vi "create.vi"(6 "enqueue (back)":T1, 7 "auto-reset? (T)":bool=TRUE, 8 "error in (no error)":errorcluster, 9 "interval (1000 ms)":u32=1000, 10 "message (\"\"=Ignore)":string, 11 "destination queue":refnum<queue>) -> (0 "error out":errorcluster, 3 "timer":refnum<class "rytimer.lvclass">)   [LabVIEW 2017, in "rytimer.lvclass"]
uses:
  rytimer.lvclass
  enqueue.ctl
  rytimer.lvclass/rytimer.ctl
  daemon.vi
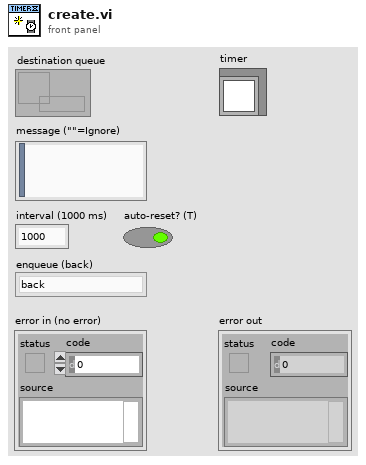
[diagram p1: front panel]
types:
  T1 = typedef "rytimer.lvclass/enqueue.ctl" = enum8{"back", "front", "back_if_absent", "front_if_absent"}
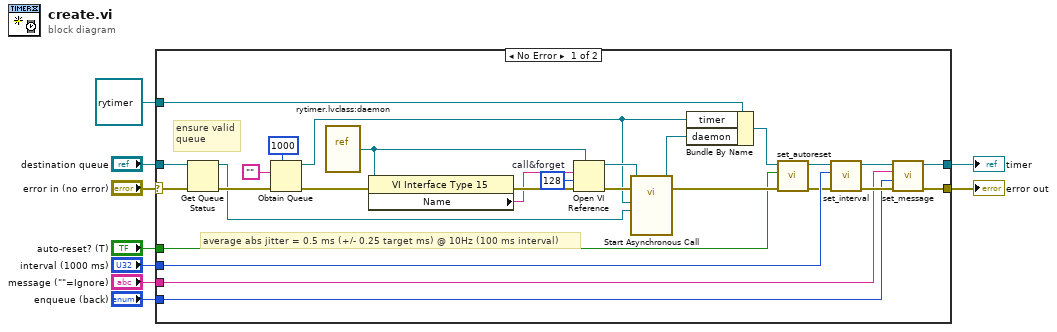
[diagram p0: block diagram]
diagram:
  n1 = case shown="No Error" "error in (no error)" {
    selector: "error in (no error)" -> [w36 w39]
    tunnel: refnum<class "rytimer.lvclass"> refnum ("timer") -> [w27 w38]
    tunnel: "interval (1000 ms)" -> [w25 _]
    tunnel: [w23 w39] -> w6
    tunnel: [w21 w38] -> w5
    tunnel: "message (\"\"=Ignore)" -> [w20 _]
    tunnel: "enqueue (back)" -> [w19 _]
    tunnel: "auto-reset? (T)" -> [w13 _]
    tunnel: "destination queue" -> [w11 _]
    frame No Error {
      w32 = 128  # call&forget
      # "average abs jitter = 0.5 ms (+/- 0.25 target ms) @ 10Hz (100 ms interval)"
      # "ensure valid\nqueue"
      n2 = Get Queue Status(queue=w11, error in (no error)=w36) -> (queue out=w10:refnum<queue>, error out=w12:errorcluster)  [unwired: 1 in, 6 out]
      n3 = Obtain Queue(max queue size (-1, unlimited)=1000, element data type="" ("Empty String Constant"), error in (no error)=w12) -> (queue out=w26:refnum<queue>, error out=w35:errorcluster)  [unwired: 2 in, 1 out]
      n4 = vi-ref "rytimer.lvclass:daemon.vi"() -> (w29:refnum<vi>)
      n5 = property class="VI Interface Type 15"(reference=w29, error in=w35) -> (error out=w34:errorcluster, "Name"=w33:string)  [unwired: 1 out]
      n6 = Open VI Reference(type specifier VI Refnum (for type only)=w29, vi path=w33, options=w32, error in (no error)=w34) -> (vi reference=w30:refnum<vi>, error out=w31:errorcluster)  [unwired: 2 in]
      n7 = call-by-ref "Start Asynchronous Call"(reference=w30, error in=w31, "queue"=w10, "timer"=w26) -> (reference out=w28:refnum<vi>, error out=w17:errorcluster)  [unwired: 10 in]
      n8 = Bundle By Name(cluster=w27, "timer"=w26, "daemon"=w28) -> (w15:refnum<class "rytimer.lvclass">)
      n9 = call "set_autoreset.vi"("error in (no error)"=w17, "auto-reset? (T)"=w13, "timer in"=w15) -> ("error out"=w16:errorcluster, "timer out"=w14:refnum<class "rytimer.lvclass">)  [unwired: 7 in]
      n10 = call "set_interval.vi"("error in (no error)"=w16, "interval (1000 ms)"=w25, "timer in"=w14) -> ("error out"=w24:errorcluster, "timer out"=w22:refnum<class "rytimer.lvclass">)  [unwired: 7 in]
      n11 = call "set_message.vi"("error in (no error)"=w24, "enqueue (back)"=w19, "message"=w20, "timer in"=w22) -> ("error out"=w23:errorcluster, "timer out"=w21:refnum<class "rytimer.lvclass">)  [unwired: 6 in]
    }
    frame Error {
    }
  }
  "error out" <- w6
  "timer" <- w5
